vi "Display Input (I32) Popup.vi"(6 "Theme":refnum<class "Theme.lvclass">, 8 "error in":errorcluster, 9 "Default Input":i32, 10 "Message":string, 11 "Graphic":T1="info") -> (0 "error out":errorcluster, 1 "Input Value":i32)   [LabVIEW 2021, in "Pop-Up.lvlib" / "Input (I32).lvclass"]
doc: "The input (I32) popup will display information to the user and wait for the operator to enter a value and click the button.\n\n<b>Note:</b> The function <b>Close Pop-Up (I32).vi</b> can be used to send a value when closing this dialog. Otherwise, use Close Pop-Up.vi to close it early.\n\nInputs:\n-Graphic [typedef combobox] - Image (PNG) for Graphic for Popup\n-Message [String] - String Variable to populate Display\n-Theme [lvclass] - the theme for the style of the popup\n-Default Input [I32] - default value for the prompt\n\nOutputs\n-Input Value [I32] - the user's entered data\n\n<b>Code Developed By:</b>\nDaniel Coons\nTechnology Service Corporation\n1983 S Liberty Drive\nBloomington, IN 47403\nPhone: 812 558-7100\ndaniel.coons@tsc.com\nwww.tsc.com/atcs"
uses:
  Input (I32).lvclass
  Graphics.ctl
  Theme/Theme.lvclass
  Input (I32).lvclass/Input (I32).ctl
  Pop-Up.lvlib
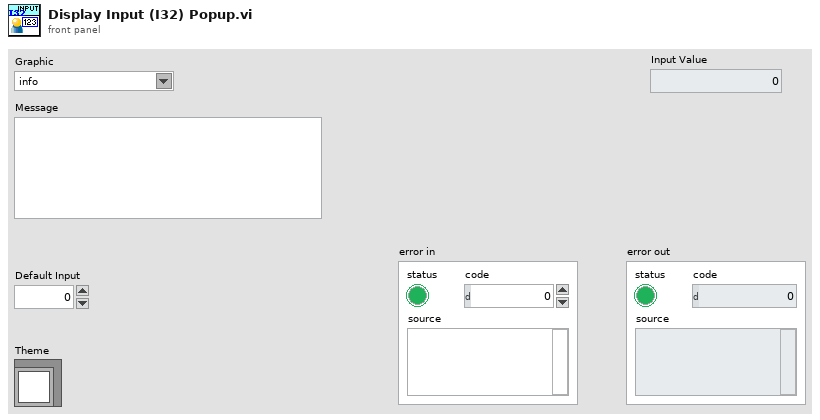
[diagram p1: front panel]
types:
  T1 = typedef "Pop-Up.lvlib/Graphics.ctl" = string
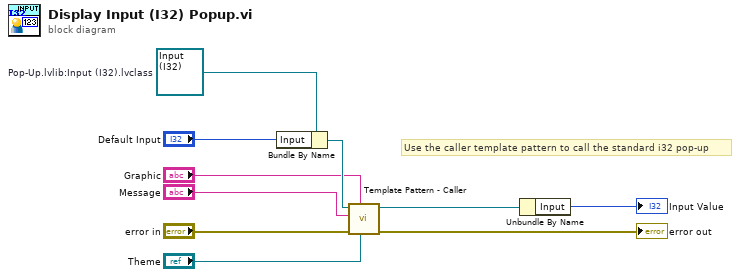
[diagram p0: block diagram]
diagram:
  w5 = refnum<class "Input (I32).lvclass"> refnum  # Pop-Up.lvlib:Input (I32).lvclass
  # "Use the caller template pattern to call the standard i32 pop-up"
  n1 = Bundle By Name(cluster=w5, "Input"="Default Input") -> (w4:refnum<class "Input (I32).lvclass">)
  n2 = call-dynamic "Template Pattern - Caller.vi"("Theme"="Theme", "standard"="Graphic", "error in (no error)"="error in", "Message"="Message", "Pop-Up in"=w4) -> ("error out"=→"error out":errorcluster, "Pop-Up out"=w9:refnum<class "Input (I32).lvclass">)  [unwired: 5 in]
  n3 = Unbundle By Name(w9) -> ("Input"=→"Input Value":i32)
